vi "Animate AppBar.vi"(8 "error in (no error)":errorcluster, 9 "Smooth?":bool=TRUE, 10 "Direction":T1, 11 "MainController in":refnum<class "MainController.lvclass">) -> (0 "error out":errorcluster, 3 "MainController out":refnum<class "MainController.lvclass">)   [LabVIEW 2012, in "Win8uiFramework.lvlib" / "MainController.lvclass"]
uses:
  MainController.lvclass
  Visibility Direction.ctl
  ViewableActor.lvclass/ViewableActor.ctl
  MainController.lvclass/MainController.ctl
  Read UI VI Ref.vi
  Read AppBar Splitter.vi
  Win8uiFramework.lvlib
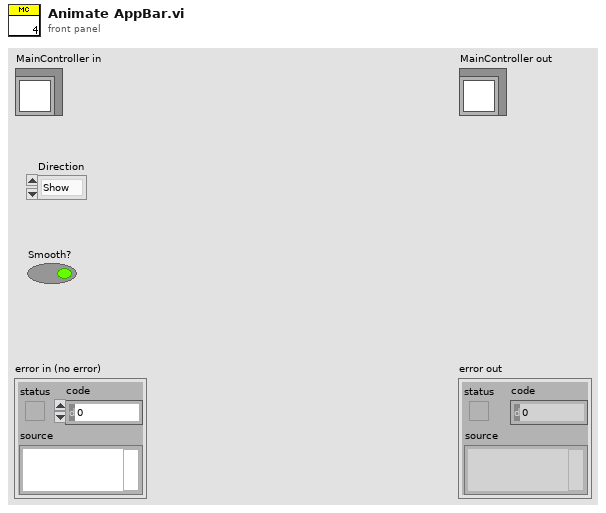
[diagram p1: front panel]
types:
  T1 = typedef "Win8uiFramework.lvlib/Visibility Direction.ctl" = enum16{"Show", "Hide"}
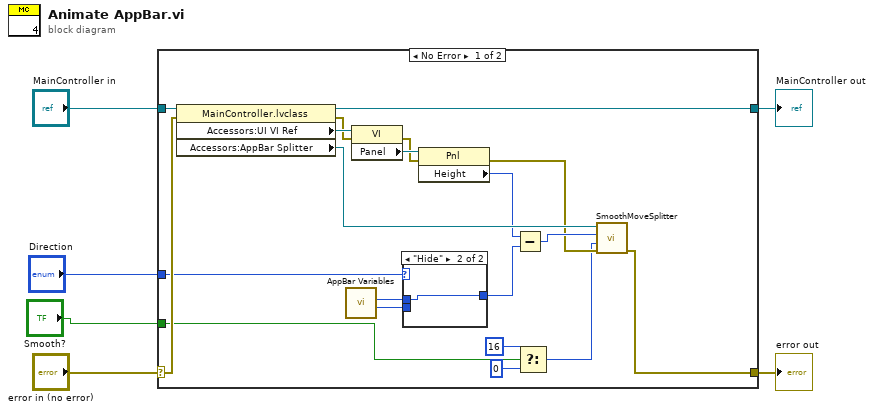
[diagram p0: block diagram]
diagram:
  n1 = case shown="No Error" "error in (no error)" {
    selector: "error in (no error)" -> [w16 w30]
    tunnel: [w15 w30] -> w5
    tunnel: [w25 w29] -> w3
    tunnel: "MainController in" -> [w26 w29]
    tunnel: "Direction" -> [w11 _]
    tunnel: "Smooth?" -> [w10 _]
    frame No Error {
      n2 = property class="MainController.lvclass"(reference=w26, error in=w16) -> (reference out=w25:refnum<class "MainController.lvclass">, error out=w19:errorcluster, "Accessors:UI VI Ref"=w23:refnum<vi>, "Accessors:AppBar Splitter"=w22:refnum<vi>)
      n3 = call "AppBar Variables.vi"() -> ("App Bar Height"=w14:i32, "App Bar Peek Height"=w12:u32)  [unwired: 10 in]
      n4 = property class="VI"(reference=w23, error in=w19) -> (error out=w18:errorcluster, "Panel"=w24:refnum<vi>)  [unwired: 1 out]
      n5 = case shown="\"Hide\"" w11 {
        tunnel: w14 -> [w27 _]
        tunnel: [w27 w28] -> w13
        tunnel: w12 -> [_ w28]
        frame "Show", Default {
        }
        frame "Hide" {
        }
      }
      n6 = property class="Pnl"(reference=w24, error in=w18) -> (error out=w17:errorcluster, "Height"=w21:u32)  [unwired: 1 out]
      n7 = Subtract(x=w21, y=w13) -> (x-y=w20:u32)
      n8 = Select(t=16 ("Steps (16)"), s=w10, f=0) -> (s? t:f=w8:i32)
      n9 = call "SmoothMoveSplitter.vi"("error in (no error)"=w17, "Steps (16)"=w8, "Position"=w20, "Splitter in"=w22) -> ("error out"=w15:errorcluster)  [unwired: 7 in]
    }
    frame Error {
    }
  }
  "error out" <- w5
  "MainController out" <- w3
